vi "FinalCleanUp.vi"(0 "Experiment State in":T1={"error"={"status"=FALSE, "code"=0, "source"=""}, "Digitizer DAQmx Tasks"={"TaskArray"=[]}, "Digitizer Settings"={"Channel Settings"=[], "Card Settings"=[]}, "Synchronization Settings"={"Synchronizer 0"="", "source terminal"="", "Synchronizer 1"="PXI1Slot2"}, "Digitizer Data"=[], "Next Shot#"="", "System Message"="", "User Shot Notes"="", "Timing Settings"={"Timing Card Settings"=[], "Timing Channel Settings"=[]}, "Timing Tasks"={"TaskArray"=[]}, "Tree"="", "Time Card/Channels"=[], "DAQ Card/Channels"=[], "Program Version"="", "RIO Settings"={"Channel Settings"=[], "Card Settings"=[]}, "RIO References"={"Reference Array"=[]}, "RIO Data"={"RIO Deleaved Data"=[], "Raw Readout"=[]}, "RIO Card/Channels"=[3, 8], "DIO Channels"=0, "DIO Settings"={"DIO Channel Array"=[]}} {"RIO Settings"."Card Settings"."Sample Rate" format="%#_3p"; "Timing Settings"."Timing Channel Settings"."FrontPanelTime" format="%.3p"; "Timing Settings"."Timing Channel Settings"."Pulse width (s)" format="%.3p"; "Timing Settings"."Timing Channel Settings"."Delay (s)" format="%.3p"; "Digitizer Settings"."Card Settings"."Global Edge Type" items=["Rising"=10280, "Falling"=10171]; "Digitizer Settings"."Card Settings"."Sample Rate" format="%#_3p"}) -> ()   [LabVIEW 2014]
doc: "-Release/clear all references\n-TO DO: Add FPGA clean up"
uses:
  Controls/ExperimentStateCluster.ctl
  Controls/DigitizerSettingsChannelSettings.ctl
  Controls/DigitizerSettingsCardSettingsArray.ctl
  Controls/DigitizerSettingsCardSettings.ctl
  Controls/TimingSettings.ctl
  Controls/TimingCardSettings.ctl
  Controls/TimingChannelSettings.ctl
  Controls/RIOSettingsExperimentStateCluster.ctl
  Controls/RIOSettingsChannelSettings.ctl
  Controls/RIOSettingsCardSettingsArray.ctl
  Controls/RIOSettingsCardSettings.ctl
  <vilib>/userdefined/High Color/nirio_resource_hc.ctl
  Controls/RIOData.ctl
  Controls/DIOChannel.ctl
  Controls/DAQmxCards.ctl
  <vilib>/FPGAPlugInAG/Dynamic/niLvFpga_Close_Dynamic.vi
  <vilib>/rvi/interface/nirviCloseFPGA/nirviCloseFPGA.xnode
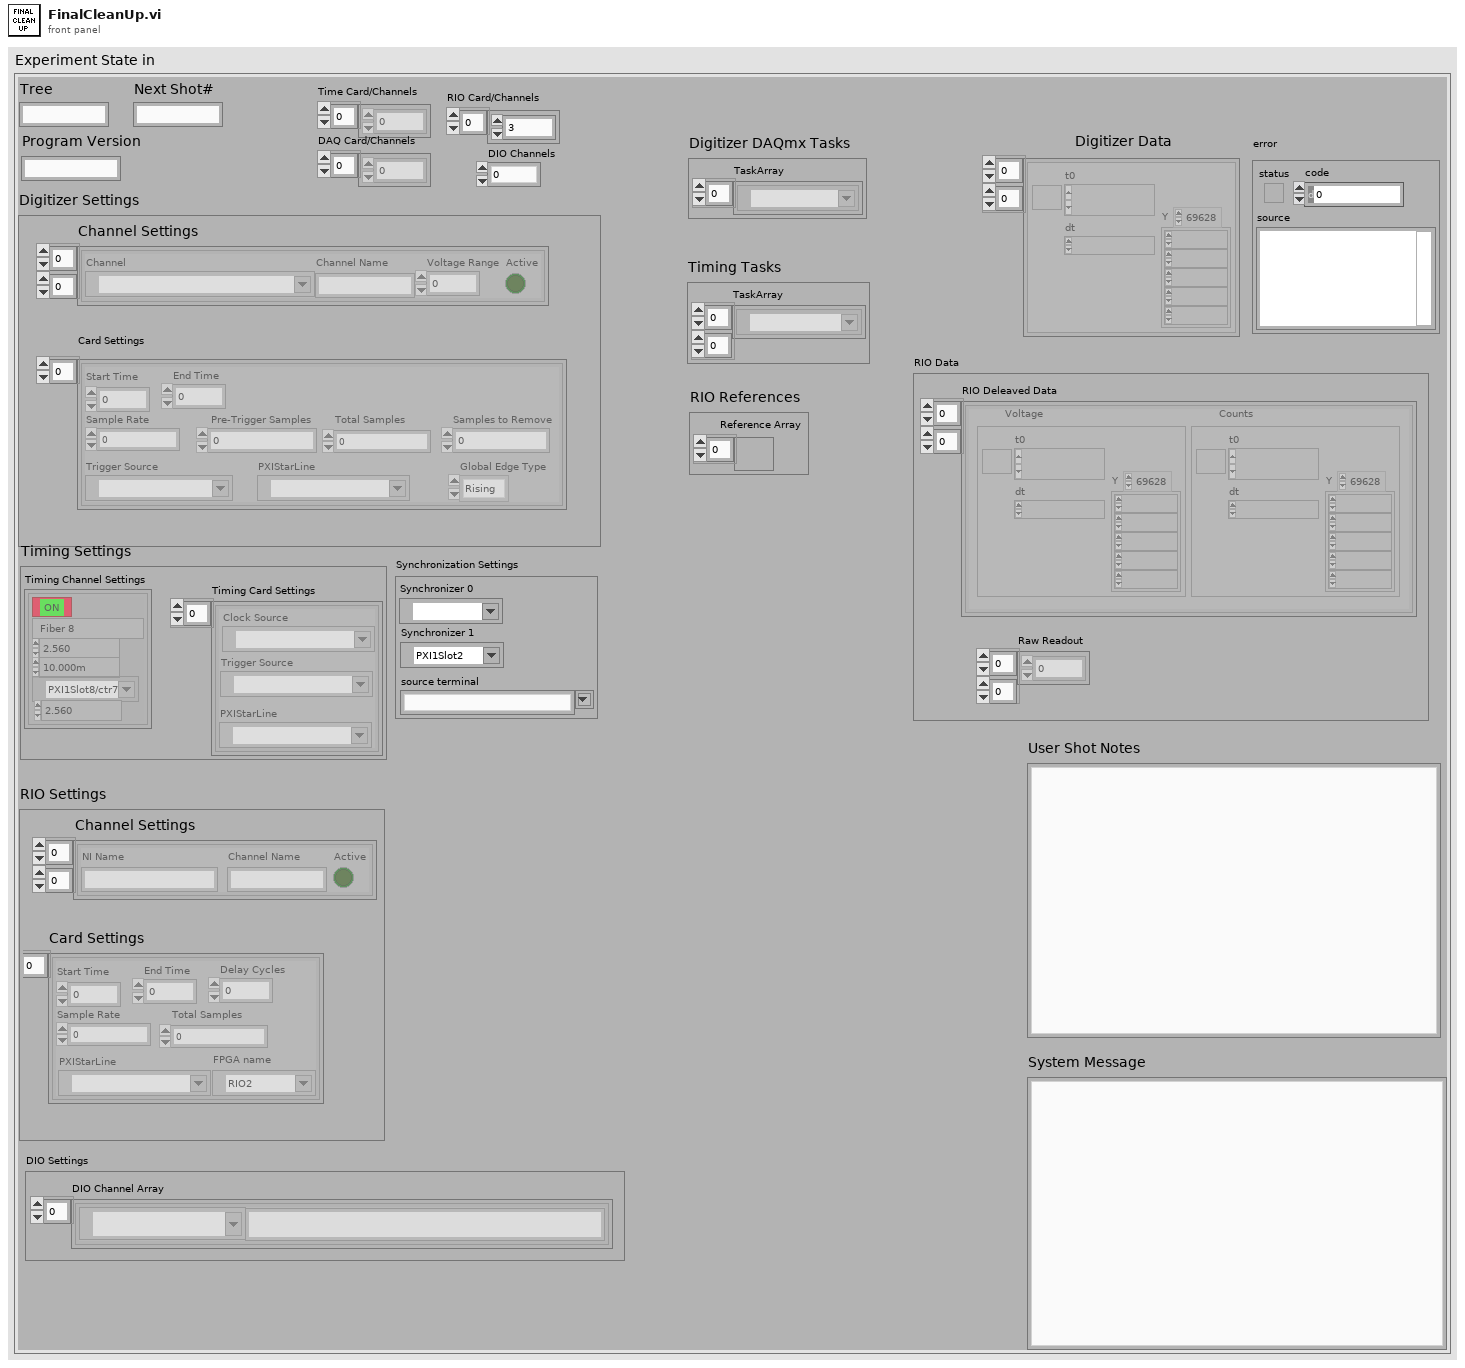
[diagram p1: front panel]
types:
  T1 = typedef "ExperimentStateCluster.ctl" = cluster{"error":errorcluster, "Digitizer DAQmx Tasks":cluster{"TaskArray":refnum<k21>[]}, "Digitizer Settings":cluster{"Channel Settings":T2[][], "Card Settings":T3}, "Synchronization Settings":cluster{"Synchronizer 0":refnum<k15>, "source terminal":string, "Synchronizer 1":refnum<k15>}, "Digitizer Data":waveform(dbl)[][], "Next Shot#":string, "System Message":string, "User Shot Notes":string, "Timing Settings":T5, "Timing Tasks":cluster{"TaskArray":refnum<k21>[][]}, "Tree":string, "Time Card/Channels":i32[], "DAQ Card/Channels":i32[], "Program Version":string, "RIO Settings":T8, "RIO References":cluster{"Reference Array":refnum<k20>[]}, "RIO Data":T13, "RIO Card/Channels":i32[], "DIO Channels":i32, "DIO Settings":cluster{"DIO Channel Array":T14[]}}
  T2 = typedef "DigitizerSettingsChannelSettings.ctl" = cluster{"Channel":tag, "Channel Name":string, "Voltage Range":dbl, "Active":bool}
  T3 = typedef "DigitizerSettingsCardSettingsArray.ctl" = T4[]
  T4 = typedef "DigitizerSettingsCardSettings.ctl" = cluster{"Start Time":dbl, "End Time":dbl, "Sample Rate":dbl, " Pre-Trigger Samples":u32, "Total Samples":i32, "Samples to Remove":u32, "Trigger Source":tag, "Global Edge Type":i32, "PXIStarLine":tag}
  T5 = typedef "TimingSettings.ctl" = cluster{"Timing Card Settings":T6[], "Timing Channel Settings":T7[][]}
  T6 = typedef "TimingCardSettings.ctl" = cluster{"Trigger Source":tag, "Clock Source":tag, "PXIStarLine":tag}
  T7 = typedef "TimingChannelSettings.ctl" = cluster{"Delay (s)":dbl, "Pulse width (s)":dbl, "Active":bool, "Channel Name":string, "counter":tag, "FrontPanelTime":dbl}
  T8 = typedef "RIOSettingsExperimentStateCluster.ctl" = cluster{"Channel Settings":T9[][], "Card Settings":T10}
  T9 = typedef "RIOSettingsChannelSettings.ctl" = cluster{"Channel Name":string, "Active":bool, "NI Name":string}
  T10 = typedef "RIOSettingsCardSettingsArray.ctl" = T11[]
  T11 = typedef "RIOSettingsCardSettings.ctl" = cluster{"Start Time":dbl, "End Time":dbl, "Sample Rate":dbl, "Total Samples":u64, "PXIStarLine":tag, "Delay Cycles":u64, "FPGA name":T12}
  T12 = typedef "nirio_resource_hc.ctl" = tag
  T13 = typedef "RIOData.ctl" = cluster{"RIO Deleaved Data":cluster{"Voltage":waveform(dbl), "Counts":waveform(i16)}[][], "Raw Readout":u64[][]}
  T14 = typedef "DIOChannel.ctl" = cluster{"Channel Name":string, "NI Name":tag}
  T15 = typedef "DAQmxCards.ctl" = tag[]
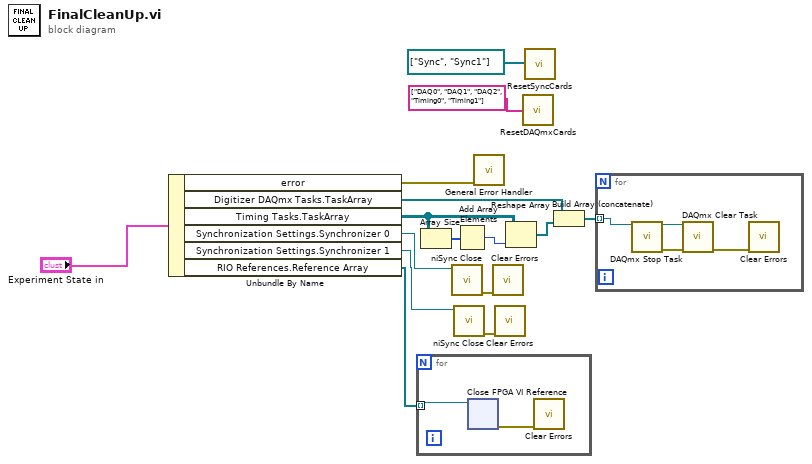
[diagram p0: block diagram]
diagram:
  n1 = Unbundle By Name("Experiment State in") -> ("error"=w10:errorcluster, "Digitizer DAQmx Tasks.TaskArray"=w11:refnum<k21>[], "Timing Tasks.TaskArray"=w15:refnum<k21>[][], "Synchronization Settings.Synchronizer 0"=w6:refnum<k15>, "Synchronization Settings.Synchronizer 1"=w4:refnum<k15>, "RIO References.Reference Array"=w2:refnum<k20>[])
  n2 = for {
    tunnel: w2 -> [w17] mode=indexing
    n3 = xnode "Close FPGA VI Reference"("FPGA VI Reference In"=w17) -> ("error out"=w16:errorcluster)  [unwired: 1 in]
    n4 = call <vilib>:"Clear Errors.vi"("error in (no error)"=w16) -> ()  [unwired: 1 in, 6 out]
  }
  n5 = Array Size(array=w15) -> (size(s)=w13:i32[])
  n6 = call <instrlib>:"niSync Close.vi"("instrument handle"=w6) -> ("error out"=w7:errorcluster)  [unwired: 1 in, 9 out]
  n7 = call <instrlib>:"niSync Close.vi"("instrument handle"=w4) -> ("error out"=w3:errorcluster)  [unwired: 1 in, 9 out]
  n8 = Add Array Elements(numeric array=w13) -> (sum=w14:i32)
  n9 = call <vilib>:"General Error Handler.vi"("error in (no error)"=w10) -> ()  [unwired: 10 in, 5 out]
  n10 = call <vilib>:"Clear Errors.vi"("error in (no error)"=w7) -> ()  [unwired: 1 in, 6 out]
  n11 = call <vilib>:"Clear Errors.vi"("error in (no error)"=w3) -> ()  [unwired: 1 in, 6 out]
  n12 = Reshape Array(w15, w14) -> (w12:refnum<k21>[])
  n13 = call "ResetDAQmxCards.vi"("Array"=T15 ["DAQ0", "DAQ1", "DAQ2", "Timing0", "Timing1"]) -> ()
  n14 = call "ResetSyncCards.vi"("Array"=refnum<k15>[] ["Sync", "Sync1"]) -> ()
  n15 = Build Array (concatenate)(w11, w12) -> (w9:refnum<k21>[])
  n16 = for {
    tunnel: w9 -> [w18] mode=indexing
    n17 = call <vilib>:"DAQmx Stop Task.vi"("task/channels in"=w18) -> ("task out"=w21:refnum<k21>, "error out"=w20:errorcluster)  [unwired: 1 in, 12 out]
    n18 = call <vilib>:"DAQmx Clear Task.vi"("task in"=w21, "error in"=w20) -> ("error out"=w19:errorcluster)  [unwired: 13 out]
    n19 = call <vilib>:"Clear Errors.vi"("error in (no error)"=w19) -> ()  [unwired: 1 in, 6 out]
  }
